vi "even or odd.vi"(5 "Numeric":u64) -> (2 "Even?":bool)   [LabVIEW 2009]
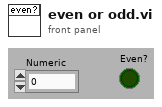
[diagram p1: front panel]
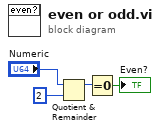
[diagram p0: block diagram]
diagram:
  n1 = Quotient & Remainder(x="Numeric", y=u64 2) -> (x-y*floor(x/y)=w2:u64)  [unwired: 1 out]
  n2 = Equal To 0?(x=w2) -> (x = 0?=→"Even?":bool)
